vi "NiXnet ConvertFramesToByteArraySinglePoint.vi"(6 "contextId":T1, 8 "error in":errorcluster, 9 "timeout (ms)":i32=-1, 10 "Request Data":T3, 11 "gRPC ID":T1) -> (0 "error out":errorcluster, 2 "Response Data":T2, 3 "gRPC ID out":T1)   [LabVIEW 2025, in "grpc-xnet_client.lvlib"]
uses:
  grpc-xnet_client.lvlib
  <vilib>/gRPC/LabVIEW gRPC Library/Shared/grpcId.ctl
  RPC Messages/nixnet_grpc_ConvertFramesToByteArraySinglePointRequest.ctl
  RPC Messages/nidevice_grpc_Session.ctl
  RPC Messages/nixnet_grpc_FrameBufferRequest.ctl
  RPC Messages/nixnet_grpc_FrameBufferRequest_frame/nixnet_grpc_FrameBufferRequest_frame.lvclass
  RPC Messages/nixnet_grpc_ConvertFramesToByteArraySinglePointResponse.ctl
  RPC Messages/nixnet_grpc_ConvertFramesToByteArraySinglePointResponse_Flat.ctl
  RPC Messages/nixnet_grpc_FrameBufferRequest_frame/nixnet_grpc_FrameBufferRequest_frame.lvclass/nixnet_grpc_FrameBufferRequest_frame.ctl
  RPC Messages/nixnet_grpc_EnetFrameRequest_type_enum/nixnet_grpc_EnetFrameRequest_type_enum.lvclass/nixnet_grpc_EnetFrameRequest_type_enum.ctl
  RPC Messages/nixnet_grpc_FrameRequest_type_enum/nixnet_grpc_FrameRequest_type_enum.lvclass/nixnet_grpc_FrameRequest_type_enum.ctl
  14035477-4c25-4107-8ed5-d0c4ef420ce5.vi
  RPC Messages/RichToFlatnidevice_grpc_Session.vi
  RPC Messages/RichToFlatnixnet_grpc_FrameBufferRequest.vi
  <vilib>/gRPC/LabVIEW gRPC Library/Shared/TranslateGrpcError.vi
  <vilib>/gRPC/LabVIEW gRPC Library/Shared/Wait On Occurrence.vi
  RPC Messages/nixnet_grpc_FrameBufferRequest_frame/GetActiveFieldIndex.vi
  RPC Messages/nixnet_grpc_FrameBufferRequest_frame/Getcan.vi
  RPC Messages/RichToFlatnixnet_grpc_FrameRequest.vi
  RPC Messages/nixnet_grpc_FrameBufferRequest_frame/Getlin.vi
  RPC Messages/nixnet_grpc_FrameBufferRequest_frame/Getflex_ray.vi
  RPC Messages/nixnet_grpc_FrameBufferRequest_frame/Getj1939.vi
  RPC Messages/nixnet_grpc_FrameBufferRequest_frame/Getenet.vi
  RPC Messages/RichToFlatnixnet_grpc_EnetFrameRequest.vi
  <vilib>/gRPC/LabVIEW gRPC Library/Shared/Is Feature Enabled.vi
  RPC Messages/nixnet_grpc_FrameRequest_type_enum/GetActiveFieldIndex.vi
  RPC Messages/nixnet_grpc_FrameRequest_type_enum/Gettype.vi
  RPC Messages/nixnet_grpc_FrameRequest_type_enum/Gettype_raw.vi
  RPC Messages/nixnet_grpc_EnetFrameRequest_type_enum/GetActiveFieldIndex.vi
  RPC Messages/nixnet_grpc_EnetFrameRequest_type_enum/Gettype.vi
  RPC Messages/nixnet_grpc_EnetFrameRequest_type_enum/Gettype_raw.vi
  <vilib>/gRPC/LabVIEW gRPC Library/Server API/Server/Get Server DLL Path.vi
  <vilib>/Utility/error.llb/Error Cluster From Error Code.vi
  RPC Messages/nixnet_grpc_EnetFrameRequest_type_enum/nixnet_grpc_EnetFrameRequest_type_enum.lvclass
  RPC Messages/nixnet_grpc_FrameRequest_type_enum/nixnet_grpc_FrameRequest_type_enum.lvclass
  <vilib>/gRPC/LabVIEW gRPC Library/grpc-lvsupport-release.lvlib
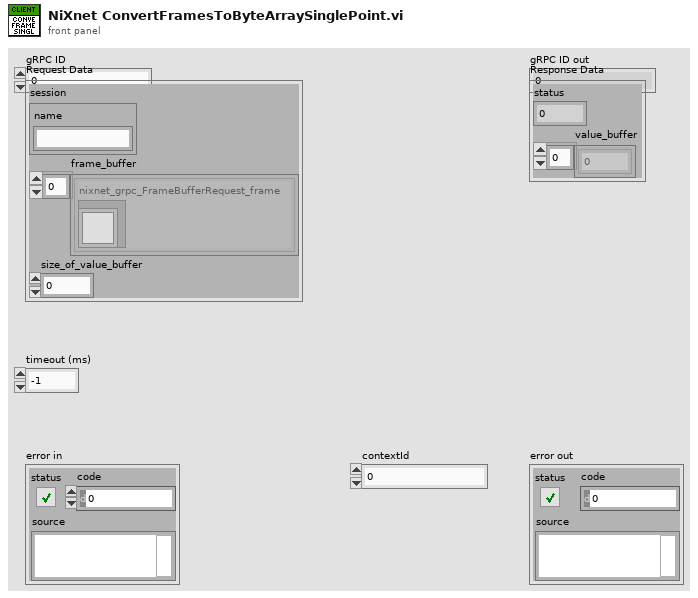
[diagram p1: front panel]
types:
  T1 = typedef "grpc-lvsupport-release.lvlib/grpcId.ctl" = u64
  T2 = typedef "grpc-xnet_client.lvlib/nixnet_grpc_ConvertFramesToByteArraySinglePointResponse.ctl" = cluster{"status":i32, "value_buffer":u8[]}
  T3 = typedef "grpc-xnet_client.lvlib/nixnet_grpc_ConvertFramesToByteArraySinglePointRequest.ctl" = cluster{"session":T4, "frame_buffer":T5[], "size_of_value_buffer":u32}
  T4 = typedef "grpc-xnet_client.lvlib/nidevice_grpc_Session.ctl" = cluster{"name":string}
  T5 = typedef "grpc-xnet_client.lvlib/nixnet_grpc_FrameBufferRequest.ctl" = cluster{"nixnet_grpc_FrameBufferRequest_frame":refnum<class "nixnet_grpc_FrameBufferRequest_frame.lvclass">}
  T6 = typedef "grpc-xnet_client.lvlib/nixnet_grpc_ConvertFramesToByteArraySinglePointResponse_Flat.ctl" = cluster{"status":i32, "value_buffer":u8[]}
  T7 = typedef "grpc-xnet_client.lvlib/nixnet_grpc_ConvertFramesToByteArraySinglePointRequest_Flat.ctl" = cluster{"session":T8, "frame_buffer":T9[], "size_of_value_buffer":u32}
  T8 = typedef "grpc-xnet_client.lvlib/nidevice_grpc_Session_Flat.ctl" = cluster{"name":string}
  T9 = typedef "grpc-xnet_client.lvlib/nixnet_grpc_FrameBufferRequest_Flat.ctl" = cluster{"nixnet_grpc_FrameBufferRequest_frame_selected_index":i32, "can":T10, "lin":T10, "flex_ray":T10, "j1939":T10, "enet":T13}
  T10 = typedef "grpc-xnet_client.lvlib/nixnet_grpc_FrameRequest_Flat.ctl" = cluster{"timestamp":u64, "identifier":u32, "nixnet_grpc_FrameRequest_type_enum_selected_index":i32, "type":T11, "type_raw":u32, "flags":T12[], "info":u32, "payload":u8[]}
  T11 = typedef "grpc-xnet_client.lvlib/nixnet_grpc_FrameType.ctl" = enum32{"FRAME_TYPE_CAN_DATA", "FRAME_TYPE_CAN_REMOTE", "FRAME_TYPE_CAN_BUS_ERROR", "FRAME_TYPE_CAN20_DATA", "FRAME_TYPE_CANFD_DATA", "FRAME_TYPE_CANFDBRS_DATA", "FRAME_TYPE_FLEX_RAY_DATA", "FRAME_TYPE_FLEX_RAY_NULL", "FRAME_TYPE_FLEX_RAY_SYMBOL", "FRAME_TYPE_LIN_DATA", "FRAME_TYPE_LIN_BUS_ERROR", "FRAME_TYPE_LIN_NO_RESPONSE", "FRAME_TYPE_J1939_DATA", "FRAME_TYPE_SPECIAL_DELAY", "FRAME_TYPE_SPECIAL_LOG_TRIGGER", "FRAME_TYPE_SPECIAL_START_TRIGGER"}
  T12 = typedef "grpc-xnet_client.lvlib/nixnet_grpc_FrameFlags.ctl" = enum32{"FRAME_FLAGS_UNSPECIFIED", "FRAME_FLAGS_FLEX_RAY_STARTUP", "FRAME_FLAGS_FLEX_RAY_SYNC", "FRAME_FLAGS_FLEX_RAY_PREAMBLE", "FRAME_FLAGS_FLEX_RAY_CH_A", "FRAME_FLAGS_FLEX_RAY_CH_B", "FRAME_FLAGS_LIN_EVENT_SLOT", "FRAME_FLAGS_TRANSMIT_ECHO"}
  T13 = typedef "grpc-xnet_client.lvlib/nixnet_grpc_EnetFrameRequest_Flat.ctl" = cluster{"nixnet_grpc_EnetFrameRequest_type_enum_selected_index":i32, "type":T14, "type_raw":u32, "device_timestamp":u64, "network_timestamp":u64, "flags_mapped":T15[], "frame_data":u8[]}
  T14 = typedef "grpc-xnet_client.lvlib/nixnet_grpc_EnetFrameType.ctl" = enum32{"ENET_FRAME_TYPE_DATA", "ENET_FRAME_TYPE_DELAY", "ENET_FRAME_TYPE_FUTURE_TIME_WAIT"}
  T15 = typedef "grpc-xnet_client.lvlib/nixnet_grpc_EnetFlags.ctl" = enum32{"ENET_FLAGS_UNSPECIFIED", "ENET_FLAGS_TRANSMIT", "ENET_FLAGS_RECEIVE", "ENET_FLAGS_NETWORK_SYNCED", "ENET_FLAGS_ERROR"}
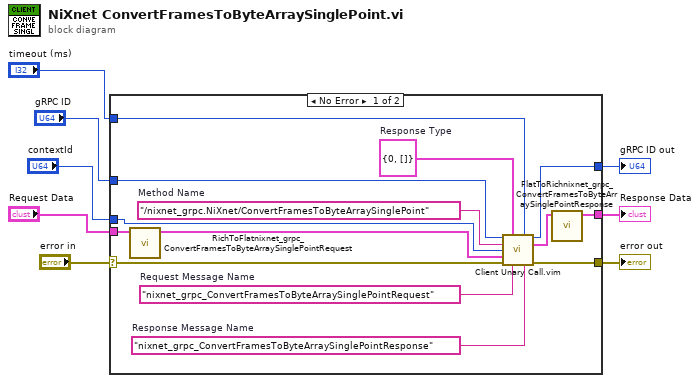
[diagram p0: block diagram]
diagram:
  n1 = case shown="No Error" "error in" {
    selector: "error in" -> [w18 w23]
    tunnel: [w17 w23] -> w7
    tunnel: "gRPC ID" -> [w16 w24]
    tunnel: [w15 w24] -> w5
    tunnel: "Request Data" -> [w12 _]
    tunnel: [w9 _] -> w3
    tunnel: "timeout (ms)" -> [w14 _]
    tunnel: "contextId" -> [w13 _]
    frame No Error {
      w19 = "nixnet_grpc_ConvertFramesToByteArraySinglePointResponse"  # Response Message Name
      w20 = "nixnet_grpc_ConvertFramesToByteArraySinglePointRequest"  # Request Message Name
      w21 = T6 {"status"=0, "value_buffer"=[]}  # Response Type
      w22 = "/nixnet_grpc.NiXnet/ConvertFramesToByteArraySinglePoint"  # Method Name
      n2 = call "RichToFlatnixnet_grpc_ConvertFramesToByteArraySinglePointRequest.vi"("InputCluster"=w12) -> ("OutputCluster"=w11:T7)  [unwired: 10 in]
      n3 = call "Client Unary Call.vim"("ClientID in"=w16, "Response Type"=w21, "timeout (ms)"=w14, "Method Name"=w22, "contextId"=w13, "Request Data"=w11, "error in"=w18, "Request Message Name"=w20, "Response Message Name"=w19) -> ("ClientID out"=w15:u64, "Response Data"=w10:T6, "error out"=w17:errorcluster)  [unwired: 4 in]
      n4 = call "FlatToRichnixnet_grpc_ConvertFramesToByteArraySinglePointResponse.vi"("InputCluster"=w10) -> ("OutputCluster"=w9:T2)  [unwired: 10 in]
    }
    frame Error {
    }
  }
  "error out" <- w7
  "gRPC ID out" <- w5
  "Response Data" <- w3
